vi "Home Axis.vi"(8 "error in (no error)":errorcluster, 11 "FINE SIM Motion Axis":refnum<class "FINE SIM Motion Axis.lvclass">) -> (0 "error out":errorcluster, 3 "FINE SIM Motion Axis":refnum<class "FINE SIM Motion Axis.lvclass">)   [LabVIEW 2022 SP3, in "FINE SIM Motion Axis.lvclass"]
uses:
  FINE SIM Motion Axis.lvclass
  FINE SIM Motion Axis.lvclass/FINE SIM Motion Axis.ctl
  TypeDefs/Homing Status.ctl
  Accessors/Write Sim Axis Data.vi
  Accessors/Read Sim Axis Data.vi
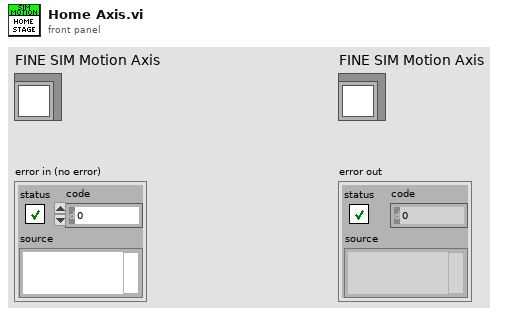
[diagram p1: front panel]
types:
  T1 = typedef "FINE SIM Motion Axis.lvclass/Axis Data.ctl" = cluster{"Axis Parameters":T2, "Time Stamp":timestamp, "Settings":T4}
  T2 = typedef "FINE SIM Motion Axis.lvclass/Axis Parameters.ctl" = cluster{"Moving":bool, "Homed":bool, "Desired Position":dbl, "Current Positon":dbl, "Current Speed":dbl, "Home Status":T3}
  T3 = typedef "FINE SIM Motion Axis.lvclass/Homing Status.ctl" = enum16{"Idle", "Inital Home Motion", "Final Home Motion", "Done Homing"}
  T4 = typedef "FINE SIM Motion Axis.lvclass/Settings.ctl" = cluster{"Axis Name":string, "Axis Settings":T5}
  T5 = typedef "FINE SIM Motion Axis.lvclass/Axis Settings.ctl" = cluster{"Speed":dbl, "Acceleration":dbl}
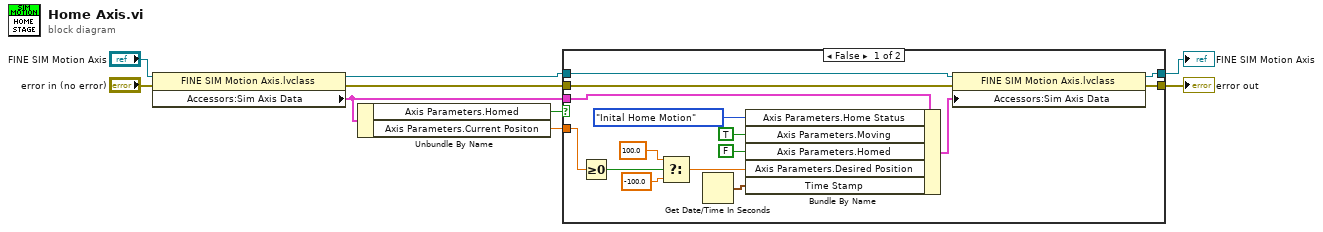
[diagram p0: block diagram]
diagram:
  n1 = property class="FINE SIM Motion Axis.lvclass"(reference="FINE SIM Motion Axis", error in="error in (no error)") -> (reference out=w9:refnum<class "FINE SIM Motion Axis.lvclass">, error out=w5:errorcluster, "Accessors:Sim Axis Data"=w7:T1)
  n2 = Unbundle By Name(w7) -> ("Axis Parameters.Homed"=w1:bool, "Axis Parameters.Current Positon"=w8:dbl)
  n3 = case shown="False" w1 {
    tunnel: w9 -> [w24 w26]
    tunnel: w8 -> [w23 _]
    tunnel: w7 -> [w21 _]
    tunnel: w5 -> [w14 w25]
    tunnel: [w13 w25] -> w4
    tunnel: [w10 w26] -> w2
    frame False {
      n4 = Greater Or Equal To 0?(x=w23) -> (x >= 0?=w22:bool)
      n5 = Select(t=100.0, s=w22, f=-100.0) -> (s? t:f=w16:dbl)
      n6 = Get Date/Time In Seconds() -> (seconds since 1Jan1904=w11:timestamp)
      n7 = Bundle By Name(cluster=w21, "Axis Parameters.Home Status"=Homing_Status."Inital Home Motion", "Axis Parameters.Moving"=TRUE, "Axis Parameters.Homed"=FALSE, "Axis Parameters.Desired Position"=w16, "Time Stamp"=w11) -> (w15:T1)
      n8 = property class="FINE SIM Motion Axis.lvclass"(reference=w24, error in=w14, "Accessors:Sim Axis Data"=w15) -> (reference out=w10:refnum<class "FINE SIM Motion Axis.lvclass">, error out=w13:errorcluster)
    }
    frame True {
    }
  }
  "error out" <- w4
  "FINE SIM Motion Axis" <- w2
